vi "init Lexer.vi"(8 "error in (no error)":errorcluster, 11 "ScintillaNET in":refnum<class "ScintillaNET.lvclass">) -> (0 "error out":errorcluster, 3 "ScintillaNET out":refnum<class "ScintillaNET.lvclass">)   [LabVIEW 2018, in "ScintillaNET.lvclass"]
uses:
  ScintillaNET.lvclass
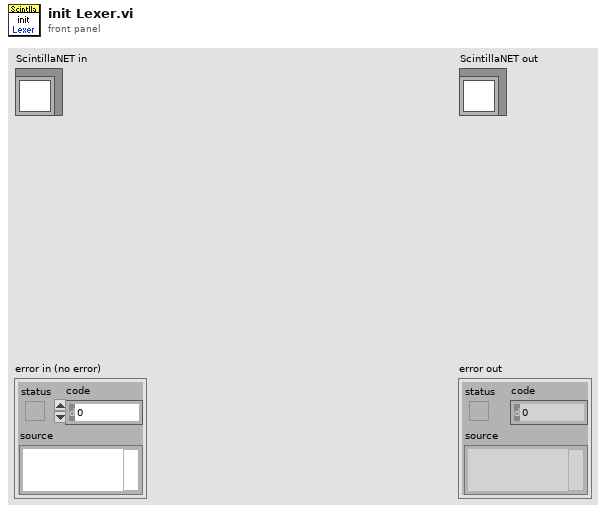
[diagram p1: front panel]
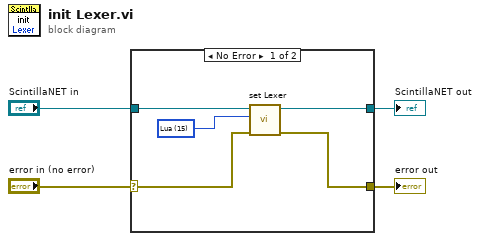
[diagram p0: block diagram]
diagram:
  n1 = case shown="No Error" "error in (no error)" {
    selector: "error in (no error)" -> [w6 w11]
    tunnel: [w7 w11] -> w3
    tunnel: [w8 w10] -> w1
    tunnel: "ScintillaNET in" -> [w9 w10]
    frame No Error {
      w5 = 15 items=["Container"=0, "Null"=1, "Python"=2, "Cpp"=3, "Html"=4, "Xml"=5, "Perl"=6, "Sql"=7, "Vb"=8, "Properties"=9, "Batch"=12, "Lua"=15, "Pascal"=18, "Ada"=20, "Lisp"=21, "Ruby"=22, "VbScript"=28, "Asm"=34, "Fortran"=36, "Css"=38, "Verilog"=56, "BlitzBasic"=66, "PureBasic"=67, "PhpScript"=69, "Smalltalk"=72, "FreeBasic"=75, "R"=86, "PowerShell"=88, "Markdown"=98, "Json"=120] ("Lexer")
      n2 = call "set Lexer.vi"("error in (no error)"=w6, "Lexer"=w5, "ScintillaNET in"=w9) -> ("error out"=w7:errorcluster, "ScintillaNET out"=w8:refnum<class "ScintillaNET.lvclass">)  [unwired: 7 in]
    }
    frame Error {
    }
  }
  "error out" <- w3
  "ScintillaNET out" <- w1
